vi "Numeric Indicator - MinMax Tracker.vi"() -> ()   [LabVIEW 2010]
doc: "Sample numeric display item."
uses:
  <vilib>/NI VeriStand/Display Template Support/Display Template Support.llb/cluster_Screen Item Settings.ctl
  <vilib>/NI VeriStand/Display Template Support/Display Template Support.llb/cluster_Graph Scale Settings.ctl
  <vilib>/NI VeriStand/Display Template Support/Display Template Support.llb/cluster_Graph Plot Settings.ctl
  NationalInstruments.VeriStand.SystemStorage
  <vilib>/NI VeriStand/Display Template Support/Display Template Support.llb/enum_Display Template Handler Minimal To Widget Msg.ctl
  <vilib>/NI VeriStand/Display Template Support/Display Template Support.llb/enum_Display Template Handler Minimal To Workspace.ctl
  <vilib>/NI VeriStand/Display Template Support/Display Template Support.llb/sub_Display Template Handler Custom.vi
  <vilib>/NI Veristand/Execution/Workspace/NI_VS Workspace ExecutionAPI.lvlib
panel:
  in  "NIVS.System Definition Root":refnum<k24>
  in  "NIVS.Gateway IP Address":string
  in  "Reset":bool
  out "Min Time":dbl format="%.2f"
  out "Max Time":dbl format="%.2f"
  out "Max":dbl format="%.2f"
  out "Min":dbl format="%.2f"
  out "Numeric":dbl format="%.2f"
  out "Label":string="Numeric"
  in  "Item.Data":T1
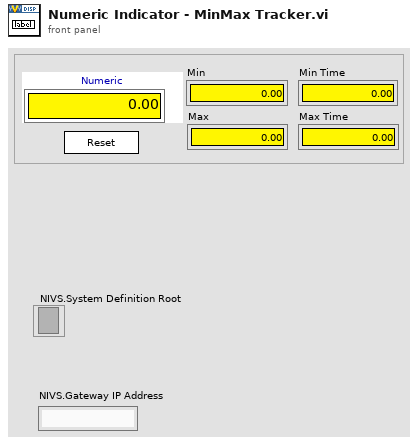
[diagram p1: front panel]
types:
  T1 = typedef "cluster_Screen Item Settings.ctl" = cluster{"Template VI":string, "Position X":i32, "Position Y":i32, "Custom":string, "Show Title Bar":bool, "ID":i32, "Always On Top":bool, "Allow Resize":bool, "Allow Minimize":bool, "Allow Close":bool, "Size to Screen":bool, "Screen.ID":i32, "State":enum16{"Normal", "New"}, "Title":string, "Window Bounds":cluster{"[0]":i16, "[1]":i16, "[2]":i16, "[3]":i16}, "Channel Ref":u64, "Unit":string, "Default Units?":bool, "Flash Limit?":bool, "Color 1":u32, "Color 2":u32, "Color 3":u32, "Color 4":u32, "Bck Color":u32, "Fore Color":u32, "Limit 1":dbl, "Limit 2":dbl, "Limit 3":dbl, "Limit 4":dbl, "Limit Mode 1":i32, "Limit Mode 2":i32, "Limit Mode 3":i32, "Limit Mode 4":i32, "Scale Precision":i32, "Scale Min":dbl, "Scale Max":dbl, "Format":i32, "Precision":i32, "Background Type":i32, "IDs":i32[], "Units":string[], "Labels":string[], "Scale Factor":dbl, "Scale Offset":dbl, "YScale Index":u32[], "XScale":T2, "YScales":T2[], "Plots":T3[], "Update Period":dbl, "History Length":dbl, "My.Ref":refnum<vi>, "Is Control?":bool, "Channel Paths":string[], "Custom Data":variant}
  T2 = typedef "cluster_Graph Scale Settings.ctl" = cluster{"Format":u8, "Precision":u8, "Fit":u8, "Label":string, "Use Default Label":bool, "Label Visible":bool, "Min":dbl, "Max":dbl}
  T3 = typedef "cluster_Graph Plot Settings.ctl" = cluster{"Bar Style":u8, "Fill To":i16, "Fill/PtColor":u32, "Line Style":u8, "Line Width":u8, "Color":u32, "Interp":u8, "Point Style":u8}
  T4 = typedef "enum_Display Template Handler Minimal To Workspace.ctl" = cluster{"Operation":enum16{"SetCustomData", "DeleteItem"}, "Data":variant}
  T5 = typedef "enum_Display Template Handler Minimal To Widget Msg.ctl" = enum16{"Stop", "LaunchConfigDialog"}
  T6 = cluster{"Node Path":string, "NodePathArray":string[]}
  T7 = typedef "NI_VS Workspace ExecutionAPI.lvlib/WorkspaceAPI.ctl" = refnum<k24>
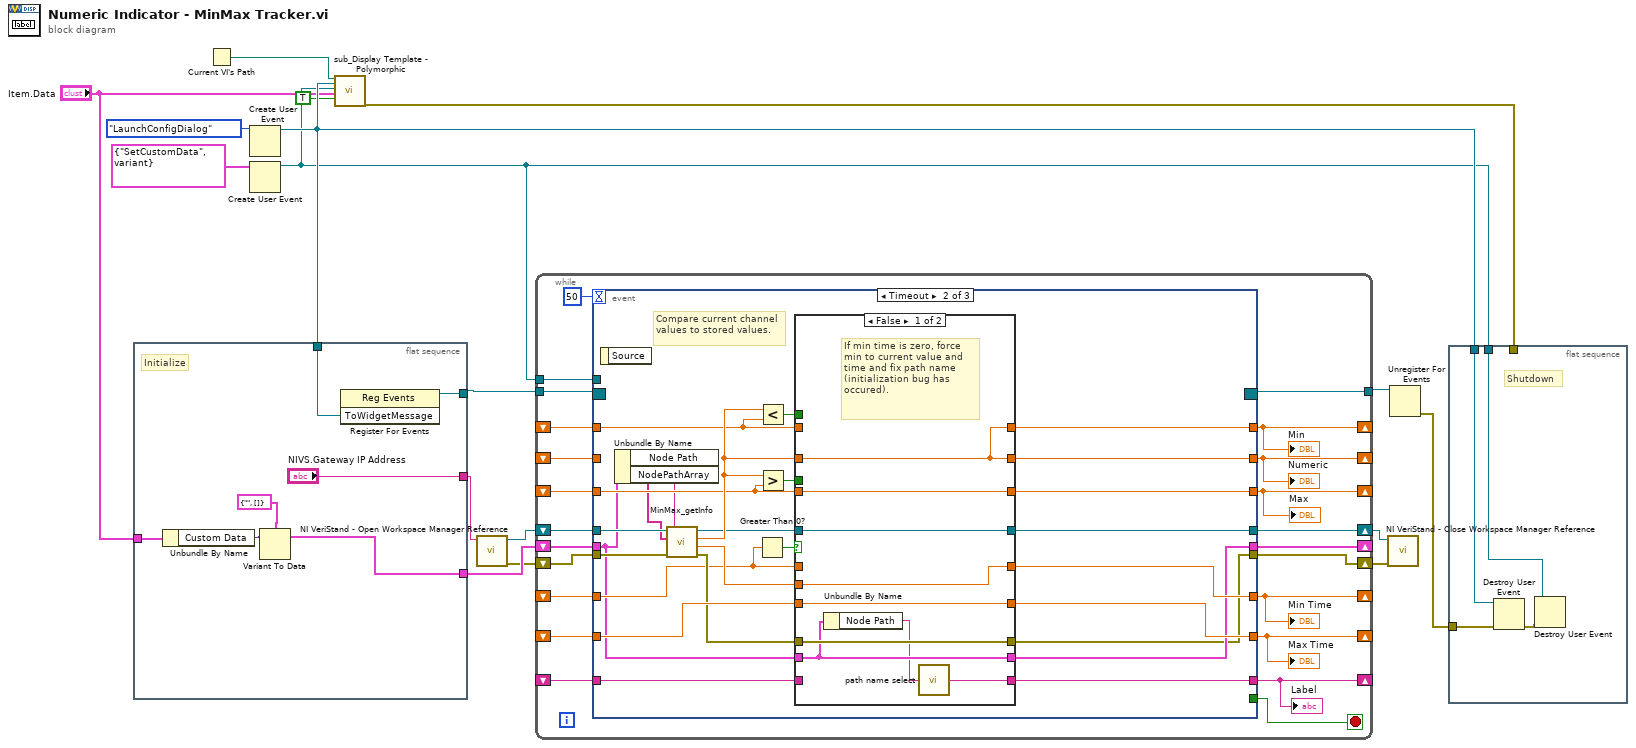
[diagram p0: block diagram]
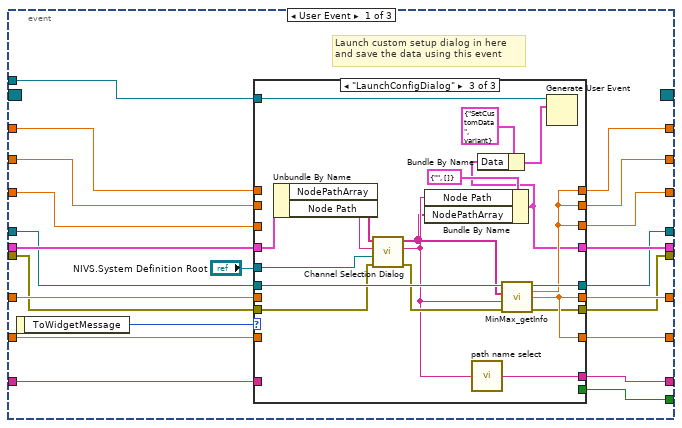
[diagram p2: hidden frame]
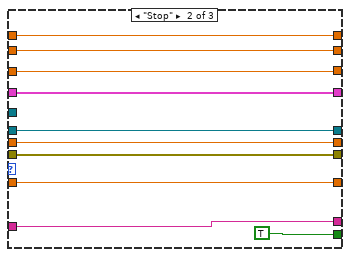
[diagram p4: hidden frame]
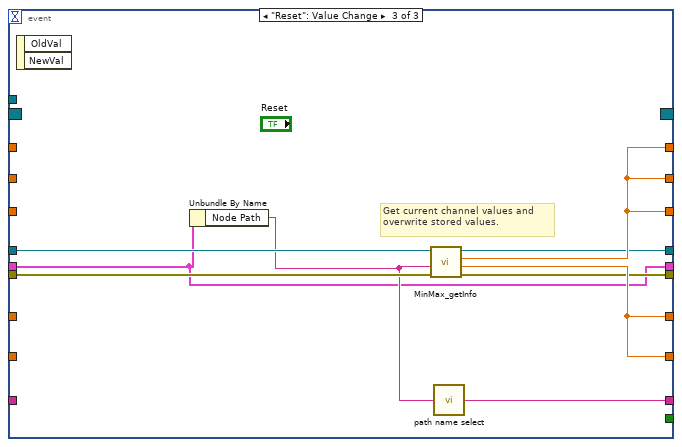
[diagram p9: hidden frame]
diagram:
  n1 = flat-sequence {
    tunnel: [w24] -> w15
    tunnel: w12 -> [w23]
    tunnel: "Item.Data" -> [w22]
    tunnel: [w20] -> w6
    tunnel: ["NIVS.Gateway IP Address"] -> w1
    frame #0 {
      # "Initialize"
      n2 = Unbundle By Name(w22) -> ("Custom Data"=w21:variant)
      n3 = Variant To Data(Variant=w21, type=T6 {"Node Path"="", "NodePathArray"=[]}) -> (data=w20:T6)  [unwired: 1 in, 1 out]
      n4 = register-events(w23) -> (reference out=w24:refnum<event-registration>)  [unwired: 2 in, 1 out]
    }
  }
  n5 = Current VI's Path() -> (path=w10:path)
  n6 = Create User Event(user event datatype=enum_Display_Template_Handler_Minimal_To_Widget_Msg."LaunchConfigDialog" ("ToWidgetMessage")) -> (user event=w12:refnum<user-event>)  [unwired: 1 in, 1 out]
  n7 = Create User Event(user event datatype=T4 {"Operation"=enum."SetCustomData", "Data"=variant} ("Data")) -> (user event=w8:refnum<user-event>)  [unwired: 1 in, 1 out]
  n8 = call-poly <vilib>:"sub_Display Template - Polymorphic.vi"("Parent.Path"=w10, "ToWidgetEvent"=w12, "ToWorkspace"=w8, "Item.Data"="Item.Data", "Resizable"=TRUE) -> ("error out"=w17:errorcluster)  [unwired: 1 in, 13 out]
  n9 = call <vilib>:"NI VeriStand - Open Workspace Manager Reference.vi"("Gateway IP Address (\"\": localhost)"=w1) -> ("error out"=w4:errorcluster, "WorkspaceManager"=w5:T7)  [unwired: 9 in]
  n10 = while {
    tunnel: w15 -> [w47]
    tunnel: [w45] -> w14
    tunnel: w8 -> [w44]
    shift-right: [w27] -> _
    shift-left: w6 -> [w43]
    shift-right: [w30] -> _
    shift-left: _ -> [w39]
    shift-right: [w40] -> _
    shift-left: _ -> [w38]
    shift-right: [w42] -> _
    shift-left: _ -> [w37]
    shift-right: [w41] -> _
    shift-left: _ -> [w36]
    shift-right: [w32] -> w3
    shift-left: w5 -> [w34]
    shift-right: [w31] -> w2
    shift-left: w4 -> [w33]
    shift-right: [w29] -> _
    shift-left: _ -> [w28]
    shift-right: [w26] -> _
    shift-left: _ -> [w25]
    stop <- w46 stop-if-true
    n11 = event shown="[1] Timeout" {
      selector: w47 -> [_ _ _]
      dyn-events: [_ _ _] -> w45
      timeout: 50 -> [_ _ _]
      tunnel: [w68 _ _] -> w46
      tunnel: w44 -> [w67 _ _]
      tunnel: [w66 w117 w206] -> w27
      tunnel: w43 -> [w65 w110 w206]
      tunnel: [w61 w123 w214] -> w42
      tunnel: [w60 w122 w214] -> w41
      tunnel: [w64 w126 w213] -> w29
      tunnel: [w63 w125 w213] -> w30
      tunnel: [w62 w124 w213] -> w40
      tunnel: w39 -> [w59 w113 _]
      tunnel: w38 -> [w58 w128 _]
      tunnel: w37 -> [w57 w112 _]
      tunnel: w36 -> [w56 w127 _]
      tunnel: w34 -> [w55 w131 w212]
      tunnel: w33 -> [w54 w130 w210]
      tunnel: [w53 w120 w211] -> w32
      tunnel: [w52 w115 w209] -> w31
      tunnel: w28 -> [w51 _ _]
      tunnel: [w50 w119 w208] -> w26
      tunnel: w25 -> [w49 w118 _]
      event User Event {
        # "Launch custom setup dialog in here\nand save the data using this event"
        n12 = event-data() -> ("ToWidgetMessage"=w69:T5)  [unwired: 1 out]
        n13 = case shown="\"LaunchConfigDialog\"" w69 {
          tunnel: [_ TRUE _] -> w68
          tunnel: w67 -> [_ _ w107]
          tunnel: [w78 w87 w90] -> w66
          tunnel: w65 -> [w78 w87 w95]
          tunnel: [w71 w80 w100] -> w64
          tunnel: [w77 w86 w100] -> w63
          tunnel: [w76 w85 w100] -> w62
          tunnel: [w75 w84 w104] -> w61
          tunnel: [w74 w83 w104] -> w60
          tunnel: w59 -> [w77 w86 _]
          tunnel: w58 -> [w76 w85 _]
          tunnel: w57 -> [w75 w84 _]
          tunnel: w56 -> [w74 w83 _]
          tunnel: w55 -> [w73 w82 w103]
          tunnel: w54 -> [w72 w81 w98]
          tunnel: [w73 w82 w102] -> w53
          tunnel: [w72 w81 w101] -> w52
          tunnel: w51 -> [w71 w80 _]
          tunnel: [w70 w79 w99] -> w50
          tunnel: w49 -> [w70 w79 _]
          tunnel: "NIVS.System Definition Root" -> [_ _ w96]
          frame Default {
          }
          frame "Stop" {
          }
          frame "LaunchConfigDialog" {
            n14 = Unbundle By Name(w95) -> ("NodePathArray"=w93:string[], "Node Path"=w94:string)
            n15 = call "Channel Selection Dialog.vi"("error in (no error)"=w98, "NIVS.System Definition Root"=w96, "NodePath"=w94, "NodePathArray"=w93) -> ("error out"=w97:errorcluster, "Selected NodePath"=w91:string, "Selected NodePathArray"=w89:string[])  [unwired: 5 in]
            n16 = Bundle By Name(cluster=T6 {"Node Path"="", "NodePathArray"=[]}, "Node Path"=w91, "NodePathArray"=w89) -> (w90:T6)
            n17 = call "path name select.vi"("In"=w91) -> ("Out"=w99:string)
            n18 = Bundle By Name(cluster=T4 {"Operation"=enum."SetCustomData", "Data"=variant} ("event data"), "Data"=w90) -> (w105:T4)
            n19 = call "MinMax_getInfo.vi"("error in (no error)"=w97, "Current Channel"=w91, "Node Path Array"=w89, "Ref In"=w103) -> ("error out"=w101:errorcluster, "System Time"=w104:dbl, "Current Value"=w100:dbl, "Ref Out"=w102:T7)  [unwired: 2 in]
            n20 = Generate User Event(user event=w107, event data cluster=w105) -> ()  [unwired: 1 in, 2 out]
          }
        }
      }
      event Timeout {
        # "Compare current channel values to stored values."
        n21 = event-data() -> ()  [unwired: 2 out]
        n22 = Unbundle By Name(w110) -> ("Node Path"=w109:string, "NodePathArray"=w108:string[])
        n23 = call "MinMax_getInfo.vi"("error in (no error)"=w130, "Current Channel"=w109, "Node Path Array"=w108, "Ref In"=w131) -> ("error out"=w116:errorcluster, "System Time"=w114:dbl, "Current Value"=w129:dbl, "Ref Out"=w121:T7)  [unwired: 2 in]
        n24 = Greater Than 0?(x=w112) -> (x > 0?=w111:bool)
        n25 = Less?(x=w129, y=w113) -> (x < y?=w133:bool)
        n26 = Greater?(x=w129, y=w128) -> (0:w132:bool)
        n27 = case shown="False" w111 {
          tunnel: w133 -> [_ w160]
          tunnel: w132 -> [_ w159]
          tunnel: w129 -> [w136 w158]
          tunnel: w113 -> [_ w157]
          tunnel: w128 -> [w139 w156]
          tunnel: w112 -> [_ w155]
          tunnel: w127 -> [w138 w154]
          tunnel: w114 -> [w137 w153]
          tunnel: [w136 w152] -> w126
          tunnel: [w136 w151] -> w125
          tunnel: [w139 w150] -> w124
          tunnel: [w137 w149] -> w123
          tunnel: [w138 w148] -> w122
          tunnel: w121 -> [w142 w147]
          tunnel: [w142 w146] -> w120
          tunnel: w110 -> [w135 w144]
          tunnel: [w141 w145] -> w119
          tunnel: w118 -> [_ w145]
          tunnel: [w135 w144] -> w117
          tunnel: w116 -> [w140 w143]
          tunnel: [w140 w143] -> w115
          frame False {
            # "If min time is zero, force min to current value and time and fix path name (initialization bug has occured)."
            n28 = Unbundle By Name(w135) -> ("Node Path"=w134:string)
            n29 = call "path name select.vi"("In"=w134) -> ("Out"=w141:string)
          }
          frame True {
            n30 = case shown="False" w160 {
              tunnel: w159 -> [w170 w197]
              tunnel: [w168 w196] -> w149
              tunnel: [w166 w195] -> w148
              tunnel: [w173 w194] -> w150
              tunnel: w158 -> [w165 w193]
              tunnel: [w171 w192] -> w151
              tunnel: w156 -> [w174 w191]
              tunnel: w157 -> [w172 _]
              tunnel: w155 -> [w169 _]
              tunnel: w154 -> [w167 w190]
              tunnel: w153 -> [w164 w189]
              tunnel: [w163 w188] -> w152
              tunnel: w147 -> [w162 w187]
              tunnel: [w161 w186] -> w146
              frame False {
                # "New min?"
                n31 = case shown="False" w170 {
                  tunnel: [w178 w184] -> w168
                  tunnel: [w177 w183] -> w166
                  tunnel: [w180 w182] -> w173
                  tunnel: w174 -> [w180 _]
                  tunnel: w172 -> [w179 w185]
                  tunnel: [w179 w185] -> w171
                  tunnel: w169 -> [w178 w184]
                  tunnel: w167 -> [w177 _]
                  tunnel: w165 -> [w176 w182]
                  tunnel: w164 -> [_ w183]
                  tunnel: [w176 w182] -> w163
                  tunnel: w162 -> [w175 w181]
                  tunnel: [w175 w181] -> w161
                  frame False {
                    # "Pass all values"
                    # "New max?"
                  }
                  frame True {
                    # "Replace max only"
                    # "New max?"
                  }
                }
              }
              frame True {
                # "New min?"
                n32 = case shown="False" w197 {
                  tunnel: [w200 w205] -> w196
                  tunnel: [w201 w205] -> w195
                  tunnel: [w202 w204] -> w194
                  tunnel: w193 -> [w199 w204]
                  tunnel: [w199 w204] -> w192
                  tunnel: w191 -> [w202 _]
                  tunnel: w190 -> [w201 _]
                  tunnel: w189 -> [w200 w205]
                  tunnel: [w199 w204] -> w188
                  tunnel: w187 -> [w198 w203]
                  tunnel: [w198 w203] -> w186
                  frame False {
                    # "Replace min only"
                    # "New max?"
                  }
                  frame True {
                    # "Replace min and max"
                    # "New max?"
                  }
                }
              }
            }
          }
        }
      }
      event "Reset": Value Change {
        # "Get current channel values and overwrite stored values."
        n33 = event-data() -> ()  [unwired: 3 out]
        n34 = Unbundle By Name(w206) -> ("Node Path"=w207:string)
        n35 = call "MinMax_getInfo.vi"("error in (no error)"=w210, "Current Channel"=w207, "Ref In"=w212) -> ("error out"=w209:errorcluster, "System Time"=w214:dbl, "Current Value"=w213:dbl, "Ref Out"=w211:T7)  [unwired: 3 in]
        n36 = call "path name select.vi"("In"=w207) -> ("Out"=w208:string)
      }
    }
    "Numeric" <- w29
    "Min" <- w30
    "Max" <- w40
    "Min Time" <- w42
    "Max Time" <- w41
    "Label" <- w26
  }
  n37 = call <vilib>:"NI VeriStand - Close Workspace Manager Reference.vi"("error in (no error)"=w2, "WorkspaceManager"=w3) -> ()  [unwired: 9 in, 1 out]
  n38 = Unregister For Events(event registration refnum=w14) -> (error out=w13:errorcluster)  [unwired: 1 in]
  n39 = flat-sequence {
    tunnel: w17 -> [_]
    tunnel: w13 -> [w217]
    tunnel: w12 -> [w218]
    tunnel: w8 -> [w215]
    frame #0 {
      # "Shutdown"
      n40 = Destroy User Event(user event=w218, error in=w217) -> (error out=w216:errorcluster)
      n41 = Destroy User Event(user event=w215, error in=w216) -> ()  [unwired: 1 out]
    }
  }
